vi "Copy Quick Drop to LabVIEW.vi"(8 "error in":errorcluster) -> (0 "error out":errorcluster)   [LabVIEW 2020, in "Scripts.lvlib"]
uses:
  Scripts.lvlib
  Quick Drop/Enclose in Structure.vi
  Quick Drop/_Enclose in Structure/Enclose in Structure.lvlib
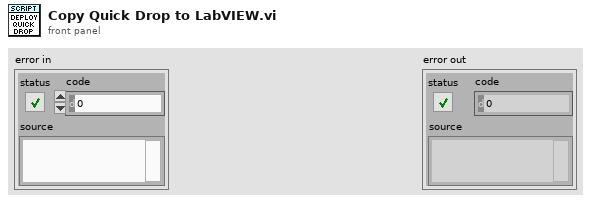
[diagram p1: front panel]
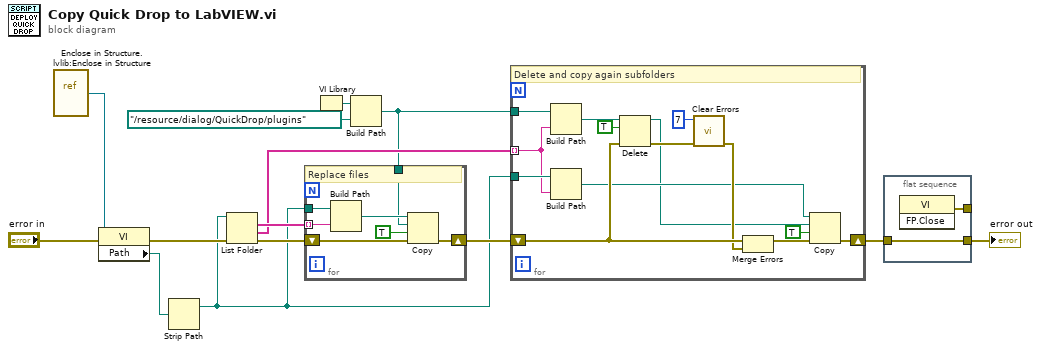
[diagram p0: block diagram]
diagram:
  n1 = vi-ref "Enclose in Structure.lvlib:Enclose in Structure.vi"() -> (w13:refnum<vi>)
  n2 = property class="VI"(reference=w13, error in="error in") -> (error out=w9:errorcluster, "Path"=w10:path)  [unwired: 1 out]
  n3 = Strip Path(path=w10) -> (stripped path=w5:path)  [unwired: 1 out]
  n4 = List Folder(path=w5, error in=w9) -> (filenames=w7:string[], folder names=w4:string[], error out=w8:errorcluster)  [unwired: 2 in, 1 out]
  n5 = VI Library() -> (path=w12:path)
  n6 = Build Path(base path=w12, name or relative path=path "../resource/dialog/QuickDrop/plugins") -> (appended path=w3:path)
  n7 = for {
    shift-right: [w17] -> w6
    shift-left: w8 -> [w18]
    tunnel: w7 -> [w20] mode=indexing
    tunnel: w5 -> [w21]
    tunnel: w3 -> [w15]
    # "Replace files"
    n8 = Build Path(base path=w21, name or relative path=w20) -> (appended path=w16:path)
    n9 = Copy(8:w18, 9:TRUE ("overwrite (F)"), 10:w15, 11:w16) -> (0:w17:errorcluster)  [unwired: 1 in, 2 out]
  }
  n10 = for {
    shift-right: [w26] -> w2
    shift-left: w6 -> [w35]
    tunnel: w5 -> [w33]
    tunnel: w4 -> [w29] mode=indexing
    tunnel: w3 -> [w30]
    # "Delete and copy again subfolders"
    n11 = Build Path(base path=w30, name or relative path=w29) -> (appended path=w28:path)
    n12 = Build Path(base path=w33, name or relative path=w29) -> (appended path=w27:path)
    n13 = Delete(path (use dialog)=w28, entire hierarchy (F)=TRUE, error in=w35) -> (deleted path=w24:path, error out=w25:errorcluster)  [unwired: 2 in, 1 out]
    n14 = call <vilib>:"Clear Errors.vi"("error in (no error)"=w25, "specific error code to clear (0: all)"=7) -> ("error out"=w34:errorcluster)  [unwired: 4 in, 1 out]
    n15 = Merge Errors(w35, w34) -> (w23:errorcluster)
    n16 = Copy(8:w23, 9:TRUE ("overwrite (F)"), 10:w24, 11:w27) -> (0:w26:errorcluster)  [unwired: 1 in, 2 out]
  }
  n17 = flat-sequence {
    tunnel: [w37] -> w1
    tunnel: w2 -> [w37]
    tunnel: [w36] -> _
    frame #0 {
      n18 = invoke class="VI" method="FP.Close"() -> (error out=w36:errorcluster)  [unwired: 3 in, 2 out]
    }
  }
  "error out" <- w1
